vi "Top Box Comms.vi"() -> ()   [LabVIEW 2019]
uses:
  RT Controls/Top Process Commands.ctl
  RT Controls/Top Command Events.ctl
  RT Controls/Top Dome Control.ctl
  RT Controls/Top Dome Status.ctl
  RT Controls/TopBox Config.ctl
  RT Controls/MainBox Idle.ctl
  <vilib>/Utility/error.llb/DialogType.ctl
  RT Controls/TopBox Json Reply.ctl
  RT Controls/TopBox Reply.ctl
  RT Controls/Top Dome Status String.ctl
  <vilib>/Utility/tcp.llb/UDP Multicast Read-Only Open.vi
panel:
  out "# elements in queue":i32
  out "error counter":u32
  out "AntWifi":bool
  out "reply":string
  out "command":string
  out "UDP data":string
  out "TopIpAddr":string
  out "TopTCPPort":u16
  out "TopUDPPort":u16
  out "top queue":refnum<queue>
  out "state":enum16{"connect", "run", "close"}(ring)
  out "TCP Data?":bool
  out "TCP error":errorcluster
  out "UDP error":errorcluster
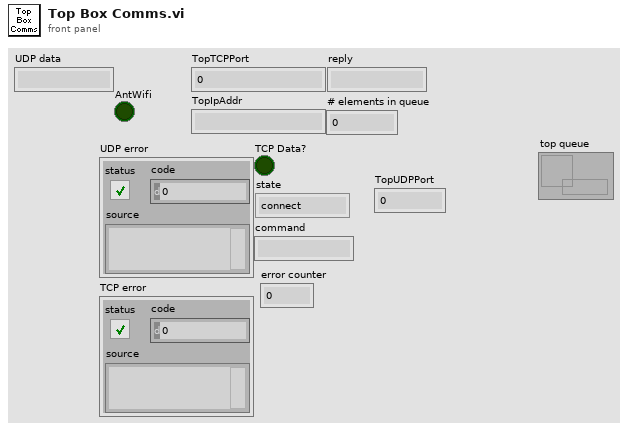
[diagram p1: front panel]
types:
  T1 = typedef "Top Process Commands.ctl" = cluster{"Command":T2, "Value":variant}
  T2 = typedef "Top Command Events.ctl" = enum16{"Idle", "FullStop", "ReadConfig", "WriteConfig", "OpenUpper", "CloseUpper", "OpenLower", "CloseLower", "SetWatchdogInt", "EnRainShutDn", "DisRainShutDn", "SetDoorMoveTO", "EnAutoShutDn", "DisAutoShutDn", "SetRevDelay", "SetRainDelay", "SyncClose", "SyncOpen"}
  T3 = typedef "TopBox Json Reply.ctl" = cluster{"reply":string, "value":T4, "error":errorcluster}
  T4 = typedef "TopBox Reply.ctl" = cluster{"TopDomeCtrl":T5, "DomeStatus":T6, "TopBoxConfig":T7}
  T5 = typedef "Top Dome Control.ctl" = cluster{"OpenLowerDoor":bool, "CloseLowerDoor":bool, "OpenMainDoor":bool, "CloseMainDoor":bool}
  T6 = typedef "Top Dome Status String.ctl" = cluster{"UpperDoorStatus":string, "LowerDoorStatus":string, "EM Button":bool, "WDTime":bool, "AutoShut":bool, "Rain":bool, "Interlock":bool, "UpperDoorEl":dbl, "LowerDoorEl":dbl, "UpperDoorEnc":u64, "LowerDoorEnc":u64}
  T7 = typedef "TopBox Config.ctl" = cluster{"WatchdogTim":i32, "RainEn":bool, "DoorMoveTO":i32, "AutoShutEn":bool, "DirRevDel":i32, "UpperClosedEnc":u64, "UpperOpenEnc":u64, "LowerClosedEnc":u64, "LowerOpenEnc":u64, "RainTim":i32, "DropoutTim":i32}
  T8 = typedef "Top Dome Status.ctl" = cluster{"UpperDoorStatus":enum16{"Ajar", "Open", "Shut", "Error"}, "LowerDoorStatus":enum16{"Ajar", "Shut", "Open", "Error"}, "EM Button":bool, "WDTime":bool, "AutoShut":bool, "Rain":bool, "Interlock":bool, "UpperDoorEl":dbl, "LowerDoorEl":dbl, "UpperDoorEnc":u64, "LowerDoorEnc":u64}
  T9 = typedef "MainBox Idle.ctl" = cluster{"EMButton":bool, "Shutdown":bool, "CloseMainDoor":bool, "OpenMainDoor":bool, "CloseLowerDoor":bool, "OpenLowerDoor":bool}
  T10 = typedef "DialogType.ctl" = u16
  T11 = cluster{"TopDomeCtrl":T5, "DomeStatus":T8, "TopBoxConfig":T7}
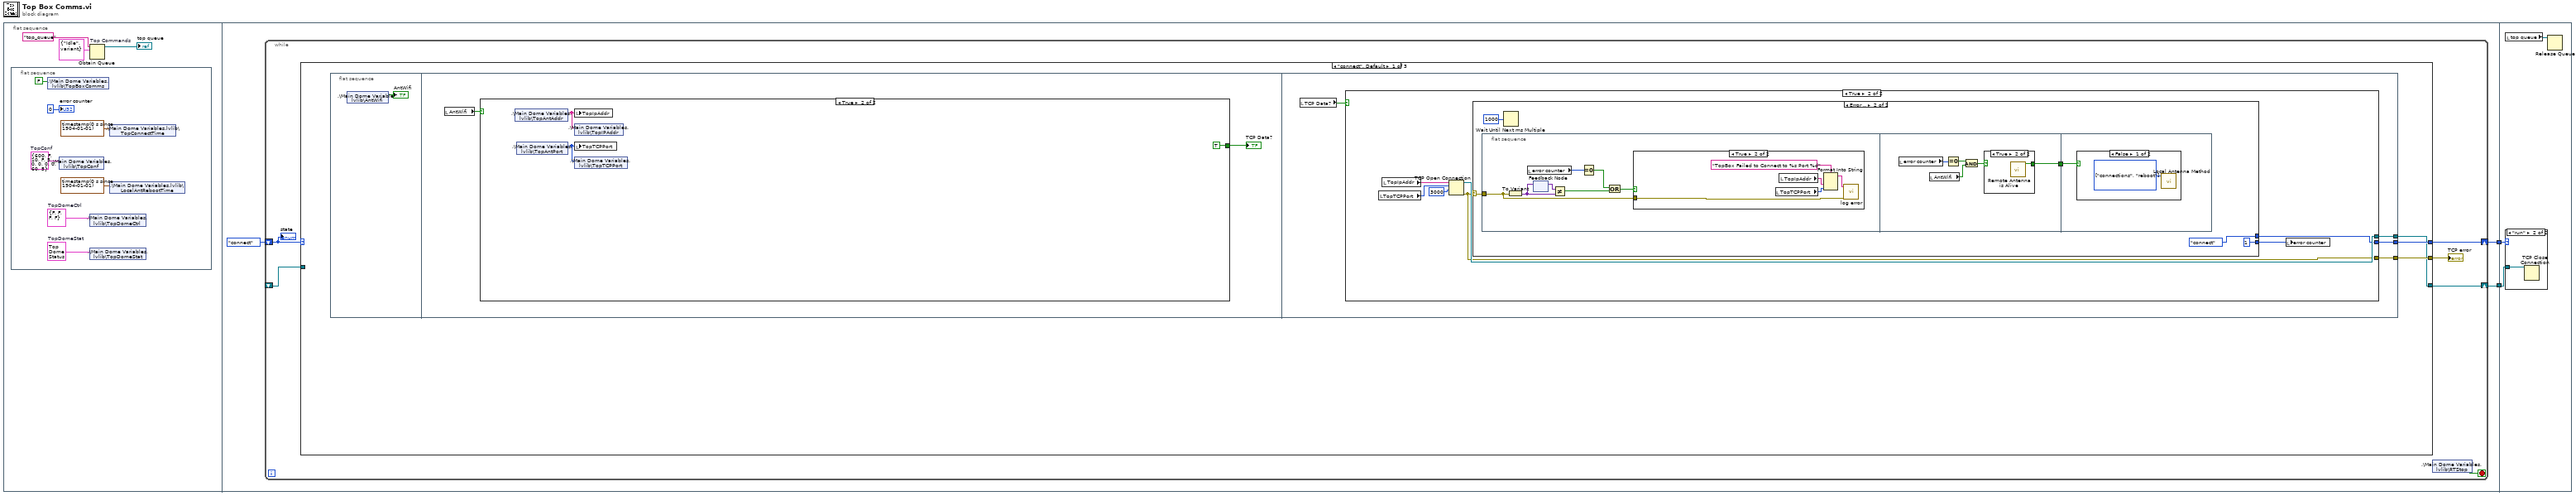
[diagram p0: block diagram]
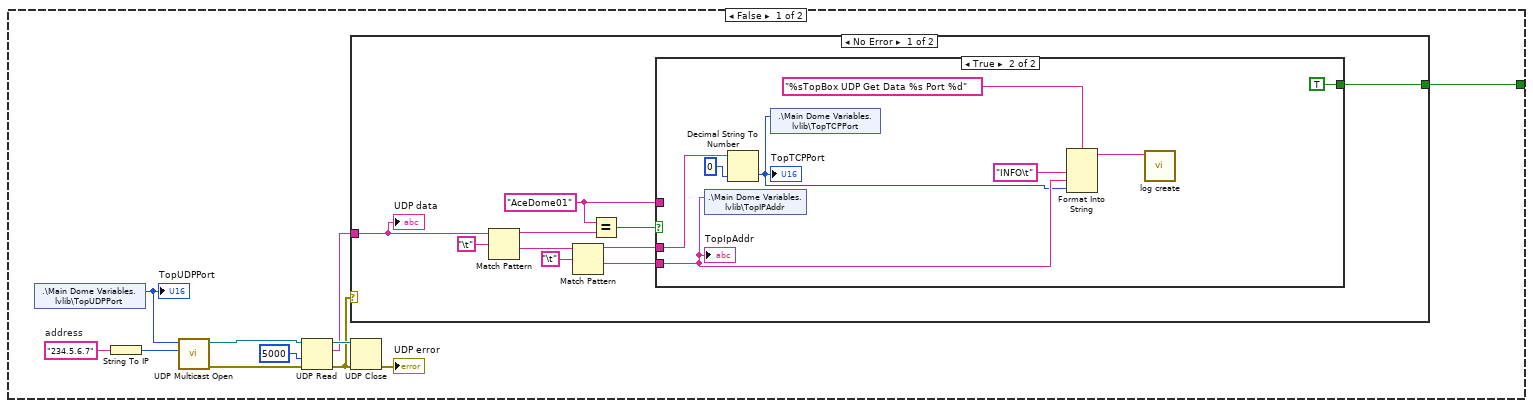
[diagram p2: hidden frame]
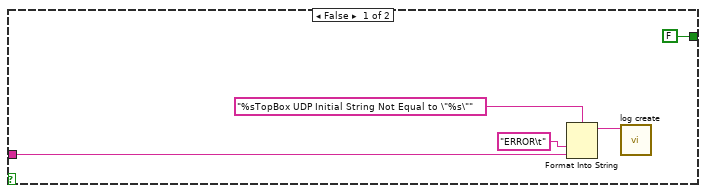
[diagram p3: hidden frame]
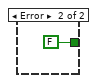
[diagram p4: hidden frame]
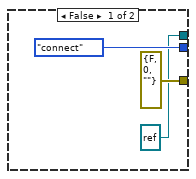
[diagram p5: hidden frame]
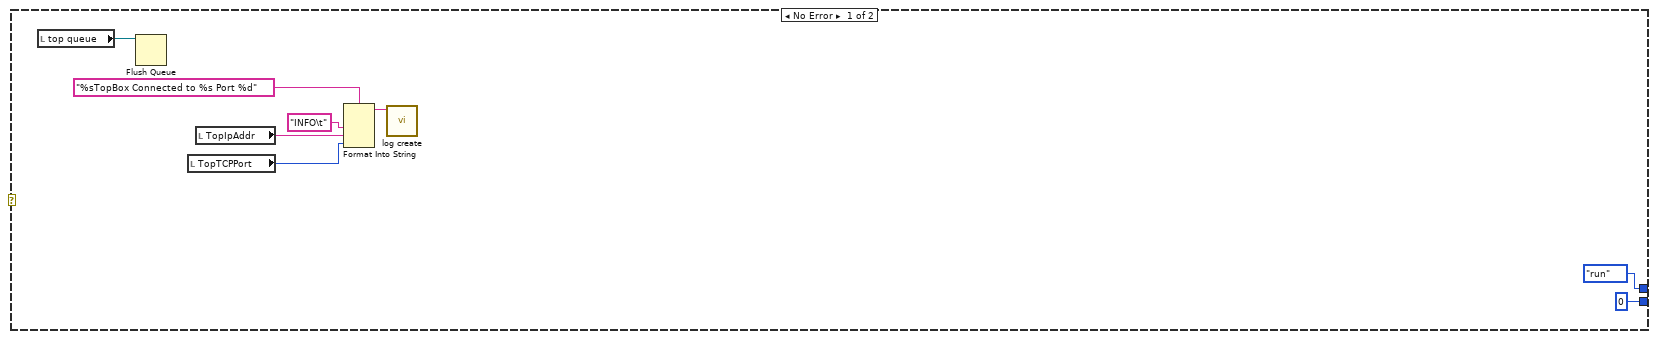
[diagram p6: hidden frame]
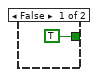
[diagram p8: hidden frame]
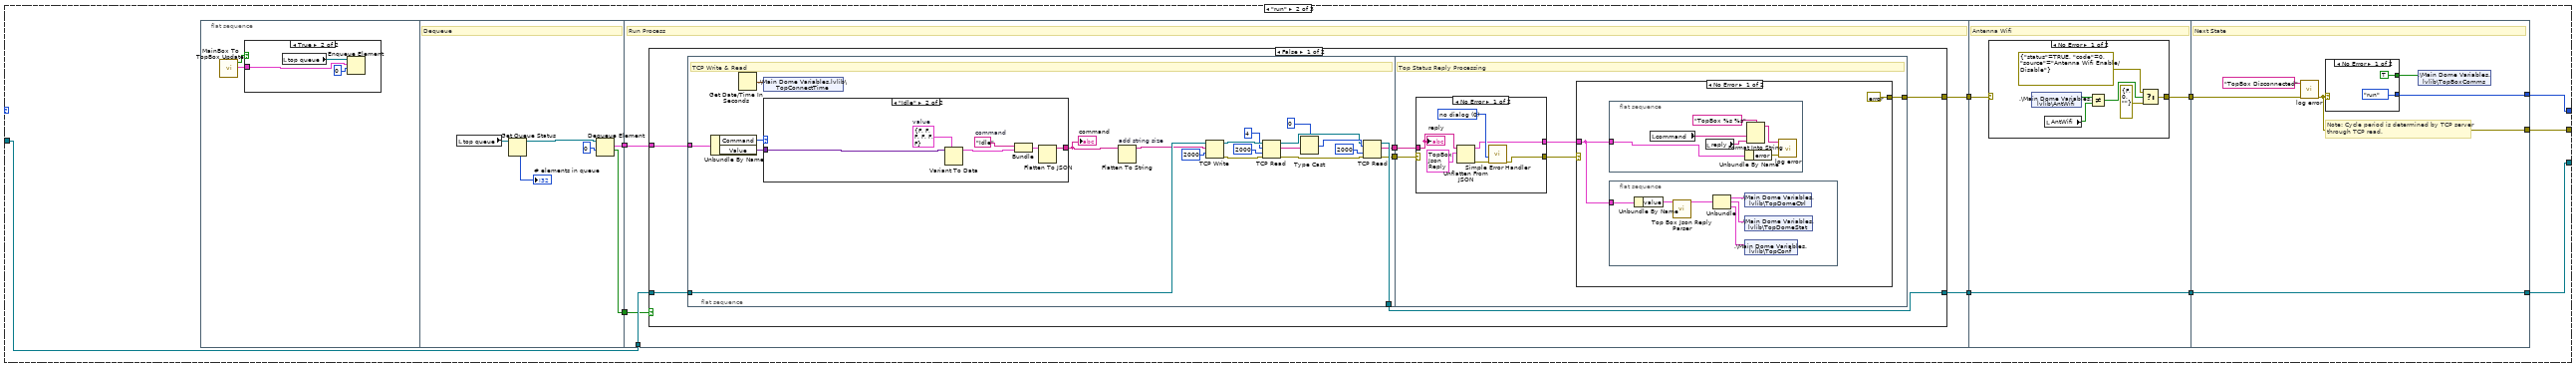
[diagram p10: hidden frame]
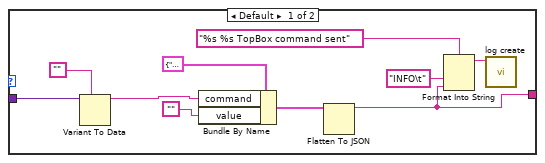
[diagram p12: hidden frame]
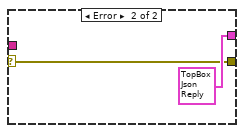
[diagram p14: hidden frame]
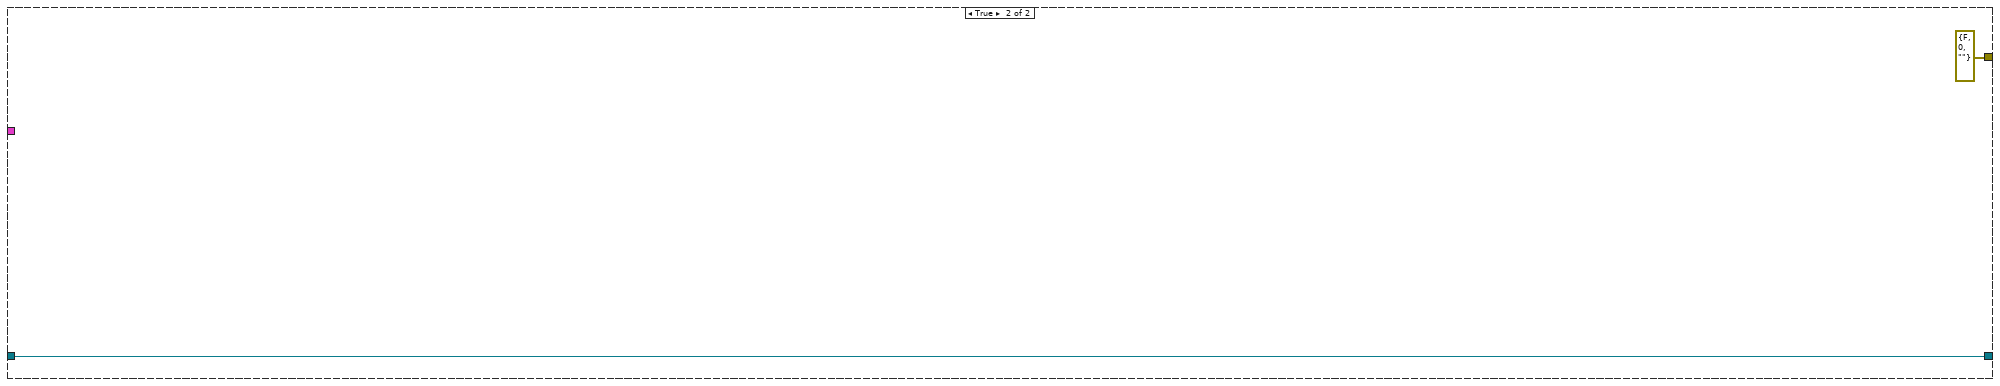
[diagram p15: hidden frame]
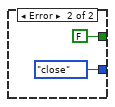
[diagram p17: hidden frame]
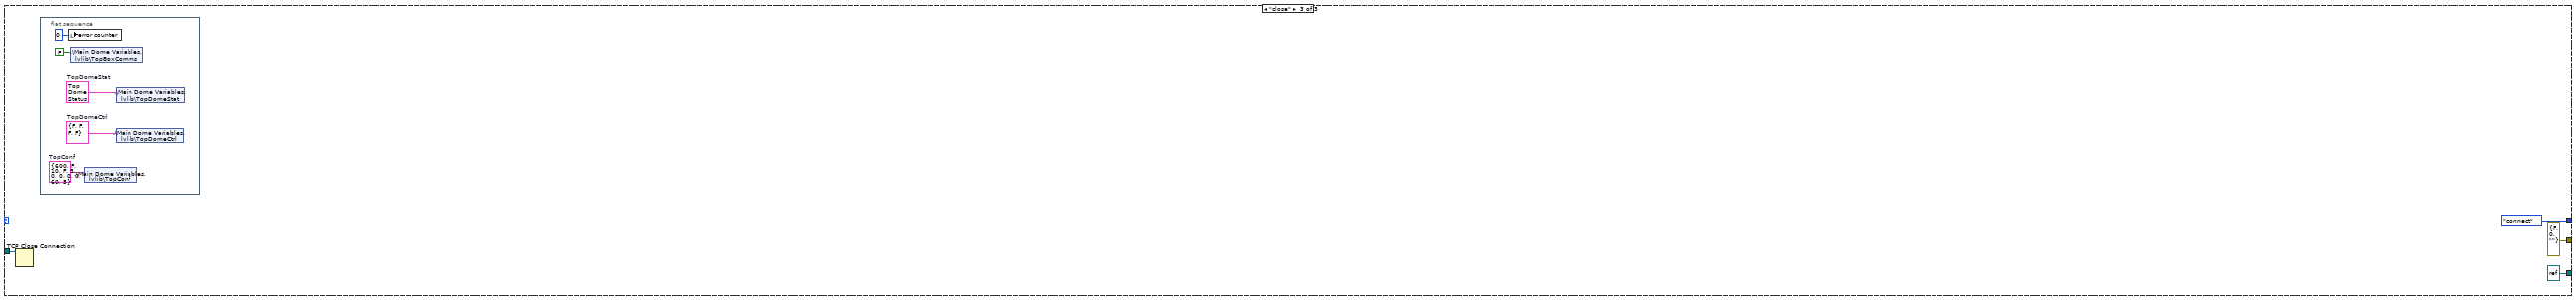
[diagram p18: hidden frame]
diagram:
  n1 = flat-sequence {
    tunnel: [w14] -> w2
    tunnel: [w13] -> w1
    tunnel: w2 -> [w243]
    tunnel: w1 -> [w244]
    frame #0 {
      n2 = flat-sequence {
        frame #0 {
          w11 = T7 {"WatchdogTim"=600, "RainEn"=FALSE, "DoorMoveTO"=10, "AutoShutEn"=FALSE, "DirRevDel"=5, "UpperClosedEnc"=0, "UpperOpenEnc"=0, "LowerClosedEnc"=0, "LowerOpenEnc"=0, "RainTim"=60, "DropoutTim"=5}  # TopConf
          w10 = T8 {"UpperDoorStatus"=enum."Ajar", "LowerDoorStatus"=enum."Ajar", "EM Button"=FALSE, "WDTime"=FALSE, "AutoShut"=FALSE, "Rain"=FALSE, "Interlock"=FALSE, "UpperDoorEl"=0.0, "LowerDoorEl"=0.0, "UpperDoorEnc"=0, "LowerDoorEnc"=0}  # TopDomeStat
          w9 = T5 {"OpenLowerDoor"=FALSE, "CloseLowerDoor"=FALSE, "OpenMainDoor"=FALSE, "CloseMainDoor"=FALSE}  # TopDomeCtrl
          n3 = shared-variable ".\\Main Dome Variables.lvlib\\TopBoxComms"(FALSE ("TopBoxComms")) -> ()  [unwired: 1 in, 1 out]
          n4 = shared-variable ".\\Main Dome Variables.lvlib\\TopConf"(w11) -> ()  [unwired: 1 in, 1 out]
          n5 = shared-variable ".\\Main Dome Variables.lvlib\\TopDomeCtrl"(w9) -> ()  [unwired: 1 in, 1 out]
          n6 = shared-variable ".\\Main Dome Variables.lvlib\\TopDomeStat"(w10) -> ()  [unwired: 1 in, 1 out]
          n7 = shared-variable ".\\Main Dome Variables.lvlib\\TopConnectTime"(timestamp(0 s since 1904-01-01) ("TopConnectTime")) -> ()  [unwired: 1 in, 1 out]
          n8 = shared-variable ".\\Main Dome Variables.lvlib\\LocalAntRebootTime"(timestamp(0 s since 1904-01-01) ("LocalAntRebootTime")) -> ()  [unwired: 1 in, 1 out]
          "error counter" <- u32 0 ("counter")
        }
      }
      n9 = Obtain Queue "Top Commands"(name (unnamed)="top_queue", element data type=T1 {"Command"=enum."Idle", "Value"=variant} ("ProcessEvents")) -> (queue out=→"top queue":refnum<queue>)  [unwired: 3 in, 2 out]
    }
    frame #1 {
      n10 = while {
        shift-right: [w18] -> w13
        shift-left: enum16{"connect", "run", "close"}."connect" -> [w20]
        shift-right: [w17] -> w14
        shift-left: _ -> [w16]
        stop <- w21 stop-if-true
        n11 = case shown="\"connect\", Default" w20 {
          tunnel: [w24 w122 errorcluster {"status"=FALSE, "code"=0, "source"=""} ("error out")] -> w19
          tunnel: [w23 w123 enum16{"connect", "run", "close"}."connect" ("f")] -> w18
          tunnel: [w22 w121 refnum<k5> refnum ("connection ID")] -> w17
          tunnel: w16 -> [_ w119 w236]
          frame "connect", Default {
            n12 = flat-sequence {
              tunnel: [w67] -> w22
              tunnel: [w68] -> w23
              tunnel: [w69] -> w24
              frame #0 {
                n13 = shared-variable ".\\Main Dome Variables.lvlib\\AntWifi"() -> (→"AntWifi":bool)  [unwired: 1 in, 1 out]
              }
              frame #1 {
                n14 = local read "AntWifi"() -> (w26:bool)
                n15 = case shown="True" w26 {
                  tunnel: [w31 TRUE] -> w27
                  frame False {
                    w30 = "234.5.6.7"  # address
                    n16 = shared-variable ".\\Main Dome Variables.lvlib\\TopUDPPort"() -> (w28:u16)  [unwired: 1 in, 1 out]
                    "TopUDPPort" <- w28
                    n17 = String To IP(1:w30) -> (0:w29:u32)
                    n18 = call-poly <vilib>:"UDP Multicast Open.vi"("multicast addr"=w29, "port"=w28) -> ("error out"=w32:errorcluster, "connection ID"=w35:refnum<k16>)  [unwired: 7 in, 1 out]
                    n19 = UDP Read(connection ID=w35, timeout ms (25000)=5000, 8:w32) -> (data out=w34:string, error out=w37:errorcluster, 3:w38:refnum<k16>)  [unwired: 1 in, 2 out]
                    n20 = case shown="No Error" w37 {
                      tunnel: w34 -> [w48 _]
                      tunnel: [w40 FALSE] -> w31
                      frame No Error {
                        w39 = "AceDome01" ("x")
                        n21 = Match Pattern(string=w48, regular expression="\t") -> (before substring=w46:string, after substring=w44:string)  [unwired: 1 in, 2 out]
                        n22 = Match Pattern(string=w44, regular expression="\t") -> (before substring=w43:string, after substring=w42:string)  [unwired: 1 in, 2 out]
                        n23 = Equal?(x=w39, y=w46) -> (x = y?=w41:bool)
                        n24 = case shown="True" w41 {
                          tunnel: w43 -> [_ w61]
                          tunnel: w42 -> [_ w55]
                          tunnel: [FALSE TRUE] -> w40
                          tunnel: w39 -> [w49 _]
                          frame False {
                            n25 = Format Into String(format string="%sTopBox UDP Initial String Not Equal to \"%s\"", "ERROR\t" ("input 1"), w49) -> (resulting string=w52:string)  [unwired: 2 in, 1 out]
                            n26 = call "log create.vi"("message"=w52) -> ()  [unwired: 11 in]
                          }
                          frame True {
                            n27 = shared-variable ".\\Main Dome Variables.lvlib\\TopIPAddr"(w55) -> ()  [unwired: 1 in, 1 out]
                            n28 = Decimal String To Number(string=w61, default (0L)=u16 0) -> (number=w54:u16)  [unwired: 1 in, 1 out]
                            "TopTCPPort" <- w54
                            n29 = shared-variable ".\\Main Dome Variables.lvlib\\TopTCPPort"(w54) -> ()  [unwired: 1 in, 1 out]
                            n30 = Format Into String(format string="%sTopBox UDP Get Data %s Port %d", "INFO\t" ("input 1"), w55, w54) -> (resulting string=w58:string)  [unwired: 2 in, 1 out]
                            n31 = call "log create.vi"("message"=w58) -> ()  [unwired: 11 in]
                            "TopIpAddr" <- w55
                          }
                        }
                        "UDP data" <- w48
                      }
                      frame Error {
                      }
                    }
                    n32 = UDP Close(connection ID=w38, 8:w37) -> (error out=→"UDP error":errorcluster)  [unwired: 1 out]
                  }
                  frame True {
                    n33 = shared-variable ".\\Main Dome Variables.lvlib\\TopAntAddr"() -> (w64:string)  [unwired: 1 in, 1 out]
                    n34 = shared-variable ".\\Main Dome Variables.lvlib\\TopAntPort"() -> (w63:u16)  [unwired: 1 in, 1 out]
                    n35 = local write "TopIpAddr"(w64) -> ()
                    n36 = shared-variable ".\\Main Dome Variables.lvlib\\TopIPAddr"(w64) -> ()  [unwired: 1 in, 1 out]
                    n37 = local write "TopTCPPort"(w63) -> ()
                    n38 = shared-variable ".\\Main Dome Variables.lvlib\\TopTCPPort"(w63) -> ()  [unwired: 1 in, 1 out]
                  }
                }
                "TCP Data?" <- w27
              }
              frame #2 {
                n39 = local read "TCP Data?"() -> (w66:bool)
                n40 = case shown="True" w66 {
                  tunnel: [errorcluster {"status"=FALSE, "code"=0, "source"=""} ("error out") w76] -> w69
                  tunnel: [enum16{"connect", "run", "close"}."connect" w77] -> w68
                  tunnel: [refnum<k5> refnum ("connection ID") w79] -> w67
                  frame False {
                  }
                  frame True {
                    n41 = local read "TopTCPPort"() -> (w73:u16)
                    n42 = local read "TopIpAddr"() -> (w74:string)
                    n43 = TCP Open Connection(address=w74, remote port or service name=w73, timeout ms (60000)=3000) -> (connection ID=w79:refnum<k5>, error out=w76:errorcluster)  [unwired: 2 in]
                    n44 = case shown="Error .." w76 {
                      selector: w76 -> [_ w90]
                      tunnel: [enum16{"connect", "run", "close"}."run" ("f") enum16{"connect", "run", "close"}."connect"] -> w77
                      tunnel: [u32 0 ("counter") u32 1] -> w75
                      frame No Error {
                        n45 = local read "top queue"() -> (w83:refnum<queue>)
                        n46 = Flush Queue(queue=w83) -> ()  [unwired: 1 in, 3 out]
                        n47 = local read "TopTCPPort"() -> (w80:u16)
                        n48 = local read "TopIpAddr"() -> (w81:string)
                        n49 = Format Into String(format string="%sTopBox Connected to %s Port %d", "INFO\t" ("input 1"), w81, w80) -> (resulting string=w86:string)  [unwired: 2 in, 1 out]
                        n50 = call "log create.vi"("message"=w86) -> ()  [unwired: 11 in]
                      }
                      frame Error {
                        n51 = flat-sequence {
                          tunnel: w90 -> [w95]
                          tunnel: [w105] -> w88
                          tunnel: w88 -> [w112]
                          frame #0 {
                            n52 = To Variant(anything=w95) -> (Variant=w94:variant)
                            n53 = local read "error counter"() -> (w99:u32)
                            n54 = feedback-in #1(w94) -> ()
                            n55 = feedback #1() -> (w93:variant)  [unwired: 1 in]
                            n56 = Not Equal?(x=w93, y=w94) -> (x != y?=w97:bool)
                            n57 = Equal To 0?(x=w99) -> (x = 0?=w98:bool)
                            n58 = Or(x=w98, y=w97) -> (x .or. y?=w96:bool)
                            n59 = case shown="True" w96 {
                              tunnel: w95 -> [_ w102]
                              frame False {
                              }
                              frame True {
                                n60 = local read "TopTCPPort"() -> (w100:u16)
                                n61 = local read "TopIpAddr"() -> (w101:string)
                                n62 = Format Into String(format string="TopBox Failed to Connect to %s Port %d", w101, w100) -> (resulting string=w104:string)  [unwired: 2 in, 1 out]
                                n63 = call "log error.vi"("error in"=w102, "message"=w104) -> ()  [unwired: 9 in, 1 out]
                              }
                            }
                          }
                          frame #1 {
                            n64 = local read "error counter"() -> (w109:u32)
                            n65 = local read "AntWifi"() -> (w108:bool)
                            n66 = Equal To 0?(x=w109) -> (x = 0?=w107:bool)
                            n67 = And(x=w107, y=w108) -> (x .and. y?=w106:bool)
                            n68 = case shown="True" w106 {
                              tunnel: [TRUE ("alive?") w111] -> w105
                              frame False {
                              }
                              frame True {
                                n69 = call "Remote Antenna is Alive.vi"() -> ("alive?"=w111:bool)  [unwired: 10 in, 1 out]
                              }
                            }
                          }
                          frame #2 {
                            n70 = case shown="False" w112 {
                              frame False {
                                w113 = enum16{"connections", "reboot"}[] [enum."connections", enum."reboot"] items=["connections", "reboot"] ("command (connections)")
                                n71 = call "Local Antenna Method.vi"("command"=w113) -> ()  [unwired: 10 in, 1 out]
                              }
                              frame True {
                              }
                            }
                          }
                        }
                        n72 = Wait Until Next ms Multiple(millisecond multiple=u32 1000) -> ()  [unwired: 1 out]
                      }
                    }
                    n73 = local write "error counter"(w75) -> ()
                  }
                }
              }
            }
          }
          frame "run" {
            n74 = flat-sequence {
              tunnel: [w133] -> w120
              tunnel: [w132] -> w118
              tunnel: [w138] -> w117
              tunnel: [w137] -> w115
              tunnel: w120 -> [w136]
              tunnel: w119 -> [w139]
              tunnel: w118 -> [w135]
              tunnel: w117 -> [w214]
              tunnel: [w213] -> w116
              tunnel: w115 -> [w215]
              tunnel: [w215] -> w114
              tunnel: [w228] -> w123
              tunnel: w116 -> [w225]
              tunnel: [w224] -> w122
              tunnel: w114 -> [w226]
              tunnel: [w226] -> w121
              frame #0 {
                n75 = call "MainBox To TopBox Update.vi"() -> ("out"=w124:T1, "enqueue?"=w125:bool)  [unwired: 10 in]
                n76 = case shown="True" w125 {
                  tunnel: w124 -> [_ w128]
                  frame False {
                  }
                  frame True {
                    n77 = local read "top queue"() -> (w126:refnum<queue>)
                    n78 = Enqueue Element(queue=w126, element=w128, timeout in ms (-1)=0) -> ()  [unwired: 1 in, 3 out]
                  }
                }
              }
              frame #1 {
                # "Dequeue"
                n79 = local read "top queue"() -> (w131:refnum<queue>)
                n80 = Get Queue Status(queue=w131) -> (queue out=w130:refnum<queue>, # elements in queue=→"# elements in queue":i32)  [unwired: 2 in, 6 out]
                n81 = Dequeue Element(queue=w130, timeout in ms (-1)=0) -> (element=w133:T1, timed out?=w132:bool)  [unwired: 1 in, 2 out]
              }
              frame #2 {
                # "Run Process"
                n82 = case shown="False" w135 {
                  tunnel: w139 -> [w143 w212]
                  tunnel: [w142 errorcluster {"status"=FALSE, "code"=0, "source"=""} ("error IO")] -> w138
                  tunnel: [w141 w212] -> w137
                  tunnel: w136 -> [w140 _]
                  frame False {
                    n83 = flat-sequence {
                      tunnel: w143 -> [w155]
                      tunnel: [w154] -> w141
                      tunnel: [w153] -> w145
                      tunnel: [w152] -> w144
                      tunnel: w140 -> [w148]
                      tunnel: [w183] -> w142
                      tunnel: w145 -> [w187]
                      tunnel: w144 -> [w186]
                      frame #0 {
                        # "TCP Write & Read"
                        n84 = Unbundle By Name(w148) -> ("Command"=w147:T2, "Value"=w146:variant)
                        n85 = Get Date/Time In Seconds() -> (seconds since 1Jan1904=w150:timestamp)
                        n86 = shared-variable ".\\Main Dome Variables.lvlib\\TopConnectTime"(w150) -> ()  [unwired: 1 in, 1 out]
                        n87 = case shown="\"Idle\"" w147 {
                          tunnel: w146 -> [w172 w182]
                          tunnel: [w167 w181] -> w149
                          frame Default {
                            n88 = Variant To Data(type="", Variant=w172) -> (data=w171:string)  [unwired: 1 in, 1 out]
                            n89 = Bundle By Name(cluster=cluster{"command":string, "value":string} {"command"="", "value"=""}, "command"=w171, "value"="") -> (w174:cluster{"command":string, "value":string})
                            n90 = Flatten To JSON(anything=w174) -> (JSON string=w167:string)  [unwired: 2 in, 1 out]
                            n91 = Format Into String(format string="%s %s TopBox command sent", "INFO\t" ("message"), w167) -> (resulting string=w169:string)  [unwired: 2 in, 1 out]
                            n92 = call "log create.vi"("message"=w169) -> ()  [unwired: 11 in]
                          }
                          frame "Idle" {
                            w178 = T9 {"EMButton"=FALSE, "Shutdown"=FALSE, "CloseMainDoor"=FALSE, "OpenMainDoor"=FALSE, "CloseLowerDoor"=FALSE, "OpenLowerDoor"=FALSE}  # value
                            w180 = "Idle"  # command
                            n93 = Variant To Data(type=w178, Variant=w182) -> (data=w177:T9)  [unwired: 1 in, 1 out]
                            n94 = Bundle("command"=w180, "value"=w177) -> (w179:cluster{"command":string, "value":T9})  [unwired: 1 in]
                            n95 = Flatten To JSON(anything=w179) -> (JSON string=w181:string)  [unwired: 2 in, 1 out]
                          }
                        }
                        "command" <- w149
                        n96 = Flatten To String "add string size"(anything=w149) -> (data string=w151:string)  [unwired: 3 in, 2 out]
                        n97 = TCP Write(connection ID=w155, data in=w151, 9:2000 ("timeout ms (25000)")) -> (connection ID out=w165:refnum<k5>, error out=w166:errorcluster)  [unwired: 1 in, 1 out]
                        n98 = TCP Read(connection ID=w165, bytes to read=4, error in (no error)=w166, 9:2000 ("timeout ms (25000)")) -> (connection ID out=w162:refnum<k5>, data out=w163:string, error out=w161:errorcluster)  [unwired: 1 in]
                        n99 = Type Cast(type=0 ("length"), x=w163) -> (*(type *) &x=w164:i32)
                        n100 = TCP Read(connection ID=w162, bytes to read=w164, error in (no error)=w161, 9:2000 ("timeout ms (25000)")) -> (connection ID out=w154:refnum<k5>, data out=w152:string, error out=w153:errorcluster)  [unwired: 1 in]
                      }
                      frame #1 {
                        # "Top Status Reply Processing"
                        n101 = case shown="No Error" w187 {
                          selector: w187 -> [_ w209]
                          tunnel: w186 -> [w208 _]
                          tunnel: [w204 w209] -> w184
                          tunnel: [w203 T3 {"reply"="", "value"={"TopDomeCtrl"={"OpenLowerDoor"=FALSE, "CloseLowerDoor"=FALSE, "OpenMainDoor"=FALSE, "CloseMainDoor"=FALSE}, "DomeStatus"={"UpperDoorStatus"="", "LowerDoorStatus"="", "EM Button"=FALSE, "WDTime"=FALSE, "AutoShut"=FALSE, "Rain"=FALSE, "Interlock"=FALSE, "UpperDoorEl"=0.0, "LowerDoorEl"=0.0, "UpperDoorEnc"=0, "LowerDoorEnc"=0}, "TopBoxConfig"={"WatchdogTim"=0, "RainEn"=FALSE, "DoorMoveTO"=0, "AutoShutEn"=FALSE, "DirRevDel"=0, "UpperClosedEnc"=0, "UpperOpenEnc"=0, "LowerClosedEnc"=0, "LowerOpenEnc"=0, "RainTim"=0, "DropoutTim"=0}}, "error"={"status"=FALSE, "code"=0, "source"=""}}] -> w185
                          frame No Error {
                            w207 = T10 0 items=["no dialog", "OK message", "continue or stop message", "OK message + warnings", "continue/stop + warnings"] ("type of dialog (OK msg:1)")
                            n102 = Unflatten From JSON(JSON string=w208, type and defaults=T3 {"reply"="", "value"={"TopDomeCtrl"={"OpenLowerDoor"=FALSE, "CloseLowerDoor"=FALSE, "OpenMainDoor"=FALSE, "CloseMainDoor"=FALSE}, "DomeStatus"={"UpperDoorStatus"="", "LowerDoorStatus"="", "EM Button"=FALSE, "WDTime"=FALSE, "AutoShut"=FALSE, "Rain"=FALSE, "Interlock"=FALSE, "UpperDoorEl"=0.0, "LowerDoorEl"=0.0, "UpperDoorEnc"=0, "LowerDoorEnc"=0}, "TopBoxConfig"={"WatchdogTim"=0, "RainEn"=FALSE, "DoorMoveTO"=0, "AutoShutEn"=FALSE, "DirRevDel"=0, "UpperClosedEnc"=0, "UpperOpenEnc"=0, "LowerClosedEnc"=0, "LowerOpenEnc"=0, "RainTim"=0, "DropoutTim"=0}}, "error"={"status"=FALSE, "code"=0, "source"=""}}) -> (value=w203:T3, error out=w206:errorcluster)  [unwired: 5 in]
                            n103 = call <vilib>:"Simple Error Handler.vi"("type of dialog (OK msg:1)"=w207, "error in (no error)"=w206) -> ("error out"=w204:errorcluster)  [unwired: 3 in, 4 out]
                            "reply" <- w208
                          }
                          frame Error {
                          }
                        }
                        n104 = case shown="No Error" w184 {
                          selector: w184 -> [_ w202]
                          tunnel: w185 -> [w189 _]
                          tunnel: [errorcluster {"status"=FALSE, "code"=0, "source"=""} ("error IO") w202] -> w183
                          frame No Error {
                            n105 = flat-sequence {
                              tunnel: w189 -> [w196]
                              frame #0 {
                                n106 = local read "command"() -> (w200:string)
                                n107 = local read "reply"() -> (w198:string)
                                n108 = Unbundle By Name(w196) -> ("error"=w197:errorcluster)
                                n109 = Format Into String(format string="TopBox %s %s" ("message"), w200, w198) -> (resulting string=w199:string)  [unwired: 2 in, 1 out]
                                n110 = call "log error.vi"("error in"=w197, "message"=w199) -> ()  [unwired: 9 in, 1 out]
                              }
                            }
                            n111 = flat-sequence {
                              tunnel: w189 -> [w195]
                              frame #0 {
                                n112 = Unbundle By Name(w195) -> ("value"=w194:T4)
                                n113 = call "Top Box Json Reply Parser.vi"("value"=w194) -> ("output cluster"=w190:T11)  [unwired: 10 in]
                                n114 = Unbundle(w190) -> ("TopDomeCtrl"=w193:T5, "DomeStatus"=w192:T8, "TopBoxConfig"=w191:T7)
                                n115 = shared-variable ".\\Main Dome Variables.lvlib\\TopDomeCtrl"(w193) -> ()  [unwired: 1 in, 1 out]
                                n116 = shared-variable ".\\Main Dome Variables.lvlib\\TopDomeStat"(w192) -> ()  [unwired: 1 in, 1 out]
                                n117 = shared-variable ".\\Main Dome Variables.lvlib\\TopConf"(w191) -> ()  [unwired: 1 in, 1 out]
                              }
                            }
                          }
                          frame Error {
                          }
                        }
                      }
                    }
                  }
                  frame True {
                  }
                }
              }
              frame #3 {
                # "Antenna Wifi"
                n118 = case shown="No Error" w214 {
                  selector: w214 -> [_ w222]
                  tunnel: [w217 w222] -> w213
                  frame No Error {
                    n119 = shared-variable ".\\Main Dome Variables.lvlib\\AntWifi"() -> (w221:bool)  [unwired: 1 in, 1 out]
                    n120 = local read "AntWifi"() -> (w220:bool)
                    n121 = Not Equal?(x=w221, y=w220) -> (x != y?=w219:bool)
                    n122 = Select(t=errorcluster {"status"=TRUE, "code"=0, "source"="Antenna Wifi Enable/Disable"}, s=w219, f=errorcluster {"status"=FALSE, "code"=0, "source"=""} ("error IO")) -> (s? t:f=w217:errorcluster)
                  }
                  frame Error {
                  }
                }
              }
              frame #4 {
                # "Note: Cycle period is determined by TCP server\nthrough TCP read."
                # "Next State"
                n123 = call "log error.vi"("error in"=w225, "message"="TopBox Disconnected") -> ("error out"=w224:errorcluster)  [unwired: 9 in]
                n124 = case shown="No Error" w224 {
                  tunnel: [enum16{"connect", "run", "close"}."run" ("f") enum16{"connect", "run", "close"}."close" ("f")] -> w228
                  tunnel: [TRUE ("TopBoxComms") FALSE ("TopBoxComms")] -> w227
                  frame No Error {
                  }
                  frame Error {
                  }
                }
                n125 = shared-variable ".\\Main Dome Variables.lvlib\\TopBoxComms"(w227) -> ()  [unwired: 1 in, 1 out]
              }
            }
          }
          frame "close" {
            n126 = TCP Close Connection(connection ID=w236) -> ()  [unwired: 2 in, 2 out]
            n127 = flat-sequence {
              frame #0 {
                w241 = T7 {"WatchdogTim"=600, "RainEn"=FALSE, "DoorMoveTO"=10, "AutoShutEn"=FALSE, "DirRevDel"=5, "UpperClosedEnc"=0, "UpperOpenEnc"=0, "LowerClosedEnc"=0, "LowerOpenEnc"=0, "RainTim"=60, "DropoutTim"=5}  # TopConf
                w240 = T8 {"UpperDoorStatus"=enum."Ajar", "LowerDoorStatus"=enum."Ajar", "EM Button"=FALSE, "WDTime"=FALSE, "AutoShut"=FALSE, "Rain"=FALSE, "Interlock"=FALSE, "UpperDoorEl"=0.0, "LowerDoorEl"=0.0, "UpperDoorEnc"=0, "LowerDoorEnc"=0}  # TopDomeStat
                w239 = T5 {"OpenLowerDoor"=FALSE, "CloseLowerDoor"=FALSE, "OpenMainDoor"=FALSE, "CloseMainDoor"=FALSE}  # TopDomeCtrl
                n128 = local write "error counter"(u32 0 ("counter")) -> ()
                n129 = shared-variable ".\\Main Dome Variables.lvlib\\TopBoxComms"(FALSE ("TopBoxComms")) -> ()  [unwired: 1 in, 1 out]
                n130 = shared-variable ".\\Main Dome Variables.lvlib\\TopConf"(w241) -> ()  [unwired: 1 in, 1 out]
                n131 = shared-variable ".\\Main Dome Variables.lvlib\\TopDomeStat"(w240) -> ()  [unwired: 1 in, 1 out]
                n132 = shared-variable ".\\Main Dome Variables.lvlib\\TopDomeCtrl"(w239) -> ()  [unwired: 1 in, 1 out]
              }
            }
          }
        }
        "TCP error" <- w19
        n133 = shared-variable ".\\Main Dome Variables.lvlib\\RTStop"() -> (w21:bool)  [unwired: 1 in, 1 out]
        "state" <- w20
      }
    }
    frame #2 {
      n134 = local read "top queue"() -> (w242:refnum<queue>)
      n135 = case shown="\"run\"" w244 {
        tunnel: w243 -> [_ w245]
        frame "connect", Default {
        }
        frame "run" {
          n136 = TCP Close Connection(connection ID=w245) -> ()  [unwired: 2 in, 2 out]
        }
      }
      n137 = Release Queue(queue=w242) -> ()  [unwired: 2 in, 3 out]
    }
  }
